vi "write out sonde row.vi"(0 "NI_report in":refnum<class "NI_report.lvclass">, 2 "Columns":i32[](array[numeric]), 3 "Column of Volume":i32, 5 "Sample Sheet Data Row Cluster":T1={"Head\nPressure"=0.0, "Depth"=0.0, "comment string"="", "Sonde Data Cluster"={"Cumulative\nVolume"=100.0, "Specific\nConductance"=2.0, "Dissolved\nOxygen"=3.0, "pH"=4.0, "ORP"=5.0, "Temp"=26.0, "Salinity"=7.0}} {"Sonde Data Cluster"."Salinity" format="%_3g"; "Sonde Data Cluster"."Temp" format="%_2g"; "Sonde Data Cluster"."ORP" format="%_4g"; "Sonde Data Cluster"."pH" format="%_4g"; "Sonde Data Cluster"."Dissolved\nOxygen" format="%_4g"; "Sonde Data Cluster"."Specific\nConductance" format="%_4g"; "Sonde Data Cluster"."Cumulative\nVolume" format="%#_4g"}, 9 "row index":i32, 11 "error in (no error)":errorcluster, 13 "start of last occupied row":cluster{"row":i32, "column":i32}) -> (4 "NI_report out":refnum<class "NI_report.lvclass">, 14 "row index out":i32, 15 "error out":errorcluster)   [LabVIEW 2016]
uses:
  <vilib>/Utility/NIReport.llb/NI_report.lvclass
  sample data row cluster.ctl
  sonde cluster.ctl
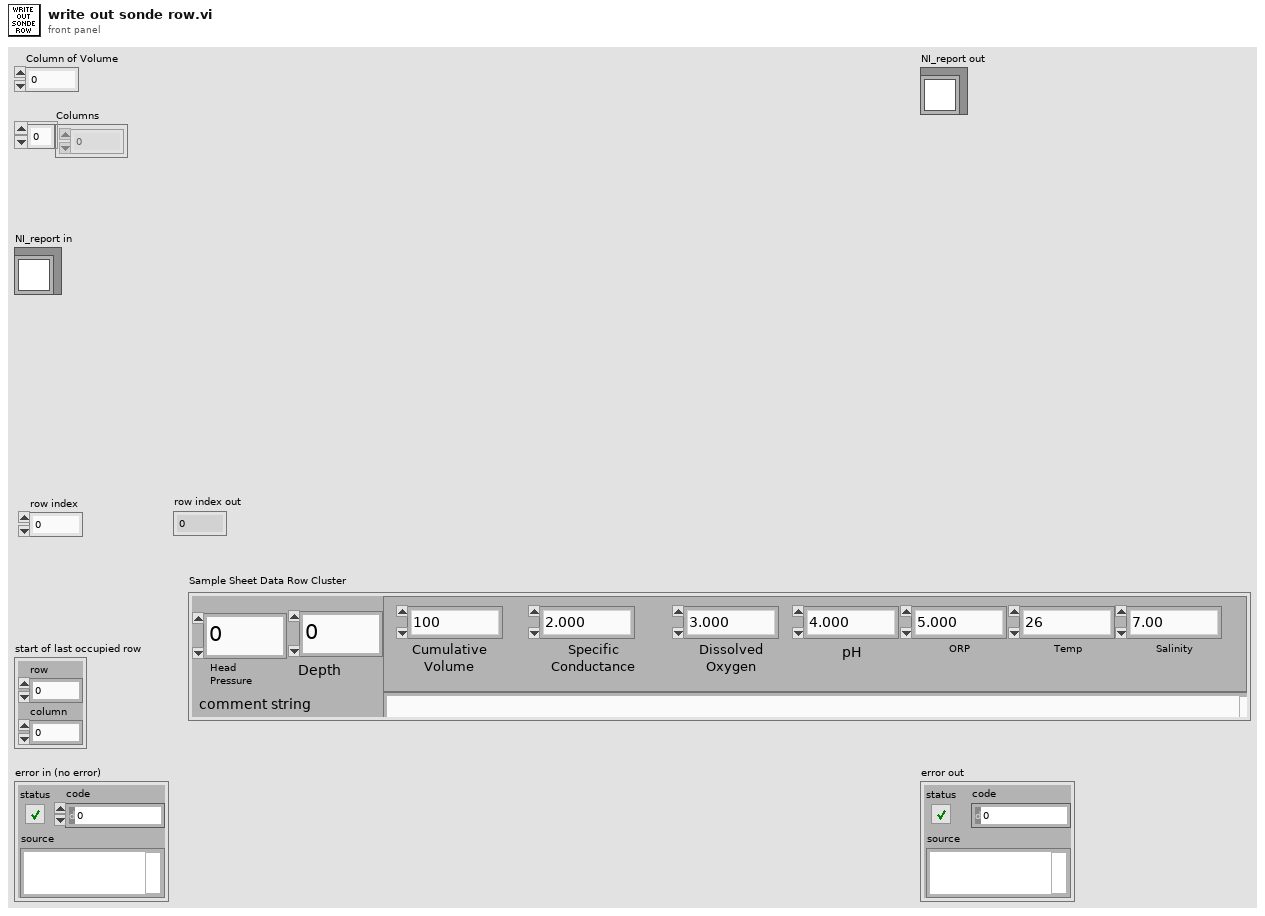
[diagram p1: front panel]
types:
  T1 = typedef "sample data row cluster.ctl" = cluster{"Head\nPressure":dbl, "Depth":dbl, "comment string":string, "Sonde Data Cluster":T2}
  T2 = typedef "sonde cluster.ctl" = cluster{"Cumulative\nVolume":dbl, "Specific\nConductance":dbl, "Dissolved\nOxygen":dbl, "pH":dbl, "ORP":dbl, "Temp":dbl, "Salinity":dbl}
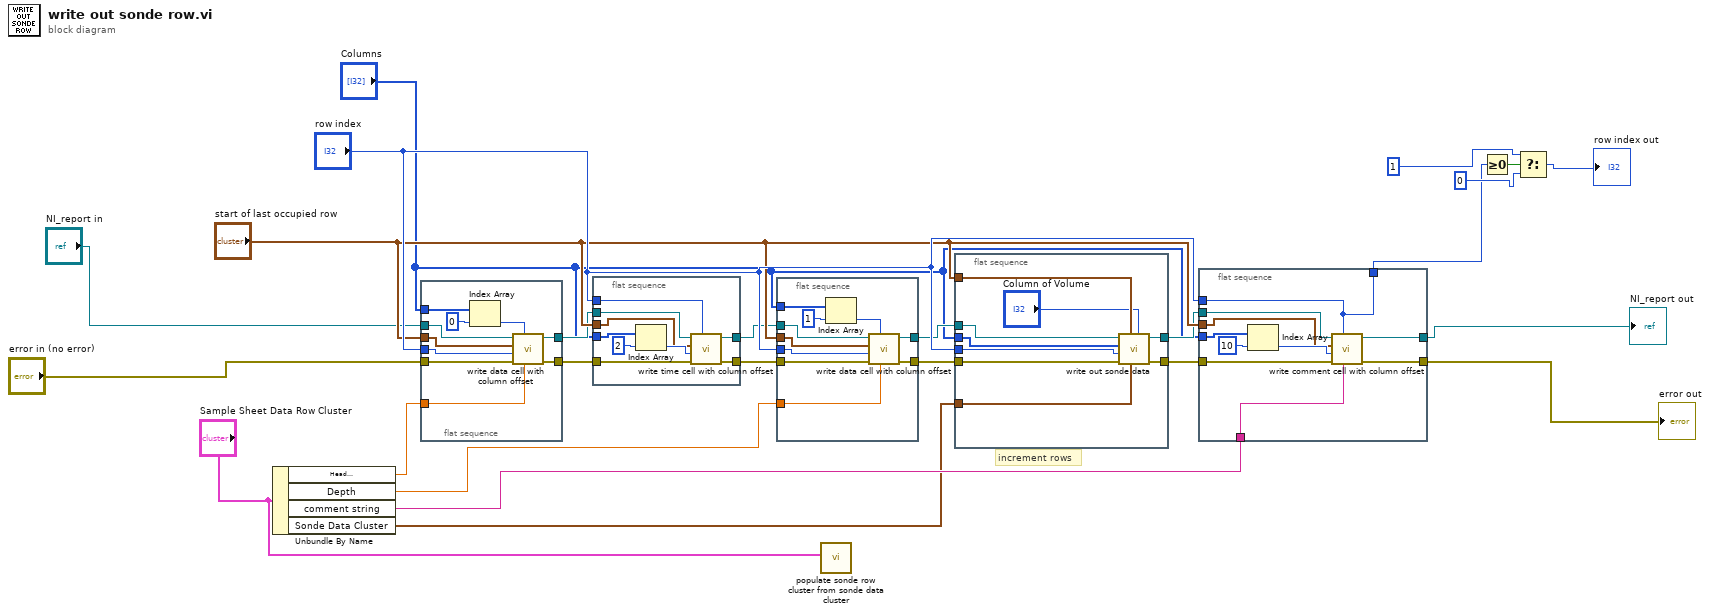
[diagram p0: block diagram]
diagram:
  # "increment rows"
  n1 = Unbundle By Name("Sample Sheet Data Row Cluster") -> ("Head\nPressure"=w10:dbl, "Depth"=w9:dbl, "comment string"=w8:string, "Sonde Data Cluster"=w7:T2)
  n2 = flat-sequence {
    tunnel: "row index" -> [w35]
    tunnel: "start of last occupied row" -> [w34]
    tunnel: [w32] -> w18
    tunnel: [w31] -> w17
    tunnel: "NI_report in" -> [w29]
    tunnel: "error in (no error)" -> [w28]
    tunnel: "Columns" -> [w27]
    tunnel: w10 -> [w26]
    frame #0 {
      n3 = Index Array(array=w27, index=0) -> (element=w33:i32)
      n4 = call "write data cell with column offset.vi"("Data Input"=w26, "data column"=w33, "error in (no error)"=w28, "row offset"=w35, "start of last occupied row"=w34, "NI_report in"=w29) -> ("error out"=w32:errorcluster, "NI_report out"=w31:refnum<class "NI_report.lvclass">)  [unwired: 4 in]
    }
  }
  n5 = flat-sequence {
    tunnel: "row index" -> [w44]
    tunnel: "start of last occupied row" -> [w41]
    tunnel: w18 -> [w40]
    tunnel: w17 -> [w39]
    tunnel: [w38] -> w16
    tunnel: [w37] -> w15
    tunnel: "Columns" -> [w36]
    frame #0 {
      n6 = Index Array(array=w36, index=2) -> (element=w43:i32)
      n7 = call "write time cell with column offset.vi"("Header offset"=w44, "error in (no error)"=w40, "time column offset"=w43, "start of last occupied row"=w41, "NI_report in"=w39) -> ("error out"=w37:errorcluster, "NI_report out"=w38:refnum<class "NI_report.lvclass">)  [unwired: 5 in]
    }
  }
  n8 = flat-sequence {
    tunnel: "row index" -> [w54]
    tunnel: [w53] -> w24
    tunnel: "start of last occupied row" -> [w52]
    tunnel: w16 -> [w51]
    tunnel: w15 -> [w50]
    tunnel: [w49] -> w14
    tunnel: "Columns" -> [w48]
    tunnel: w9 -> [w45]
    frame #0 {
      n9 = Index Array(array=w48, index=1) -> (element=w46:i32)
      n10 = call "write data cell with column offset.vi"("Data Input"=w45, "data column"=w46, "error in (no error)"=w50, "row offset"=w54, "start of last occupied row"=w52, "NI_report in"=w51) -> ("error out"=w53:errorcluster, "NI_report out"=w49:refnum<class "NI_report.lvclass">)  [unwired: 4 in]
    }
  }
  n11 = call "populate sonde row cluster from sonde data cluster.vi"("Sample Sheet Data Row Cluster"="Sample Sheet Data Row Cluster") -> ()  [unwired: 8 in, 3 out]
  n12 = flat-sequence {
    tunnel: "row index" -> [w63]
    tunnel: w24 -> [w62]
    tunnel: "Columns" -> [w61]
    tunnel: "start of last occupied row" -> [w60]
    tunnel: [w59] -> w21
    tunnel: [w58] -> w19
    tunnel: w14 -> [w57]
    tunnel: w7 -> [w55]
    frame #0 {
      n13 = call "write out sonde data.vi"("data column offset"="Column of Volume", "Sonde Data Cluster"=w55, "start of last occupied row"=w60, "error in (no error)"=w62, "Row Offset"=w63, "Header data columns"=w61, "NI_report in"=w57) -> ("error out"=w59:errorcluster, "NI_report out"=w58:refnum<class "NI_report.lvclass">)  [unwired: 3 in]
    }
  }
  n14 = flat-sequence {
    tunnel: "row index" -> [w64]
    tunnel: "Columns" -> [w71]
    tunnel: "start of last occupied row" -> [w70]
    tunnel: [w69] -> w22
    tunnel: w21 -> [w68]
    tunnel: [w67] -> w20
    tunnel: w19 -> [w66]
    tunnel: w8 -> [w65]
    tunnel: [w64] -> w3
    frame #0 {
      n15 = Index Array(array=w71, index=10) -> (element=w73:i32)
      n16 = call "write comment cell with column offset.vi"("comment string"=w65, "Row offset"=w64, "error in (no error)"=w68, "comment column offset"=w73, "start of last occupied row"=w70, "NI_report in"=w66) -> ("error out"=w69:errorcluster, "NI_report out"=w67:refnum<class "NI_report.lvclass">)  [unwired: 4 in]
    }
  }
  n17 = Greater Or Equal To 0?(x=w3) -> (x >= 0?=w6:bool)
  n18 = Select(t=1, s=w6, f=0) -> (s? t:f=→"row index out":i32)
  "error out" <- w22
  "NI_report out" <- w20
